vi "Img_Bird_eye_view.vi"(6 "parameters":T1={"P1"={"x"=970, "y"=485}, "P2"={"x"=0, "y"=750}, "Alfa"=6.0}, 8 "error in (no error)":errorcluster, 10 "Image Name":string="myimg", 11 "img annotation in":T2(plugin-control)) -> (0 "error out":errorcluster, 2 "img_corrected":T2(plugin-control), 3 "img annotation out":T2)   [LabVIEW 2021, in "Framework_lib.lvlib"]
uses:
  QMH/Framework_lib.lvlib
  <vilib>/vision/Image Controls.llb/IMAQ Image.ctl
  <vilib>/vision/NI_Vision_Development_Module.lvlib
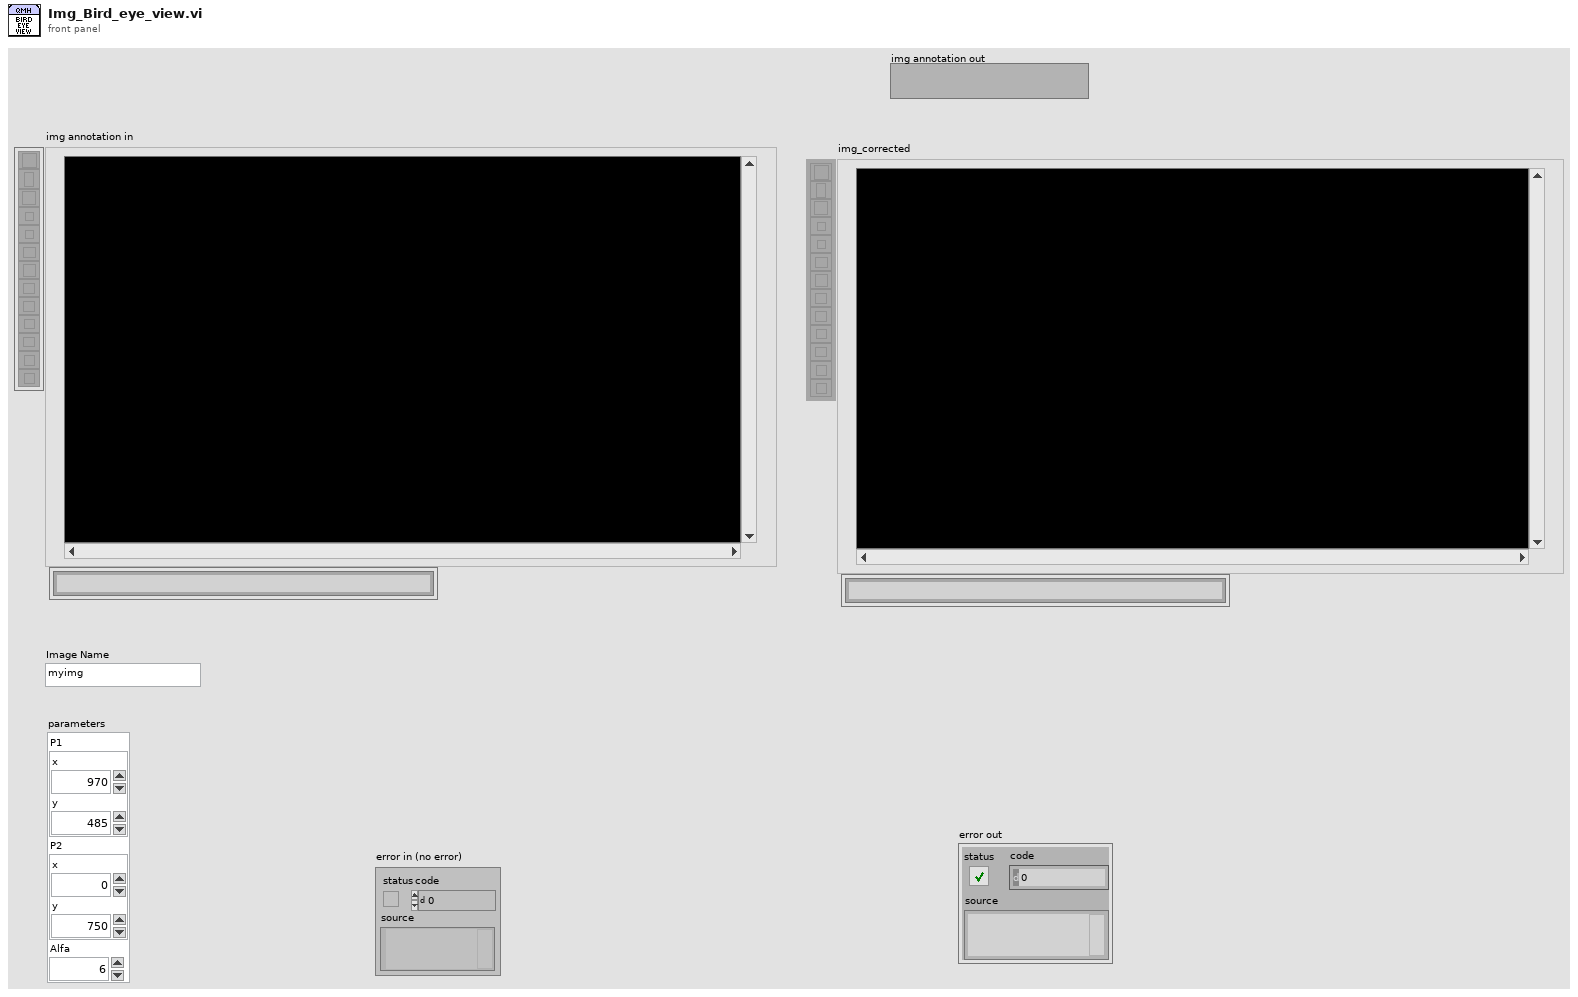
[diagram p1: front panel]
types:
  T1 = cluster{"P1":cluster{"x":i16, "y":i16}, "P2":cluster{"x":i16, "y":i16}, "Alfa":dbl}
  T2 = typedef "IMAQ Image.ctl" = refnum<image>
  T3 = typedef "Image Type" = u32
  T4 = enum32{"Zero Order", "Bilinear", "Quadratic", "Cubic", "Bilinear Fixed"}
  T5 = cluster{"Interpolation Type":enum32{"Zero Order", "Bilinear", "Quadratic", "Cubic", "Bilinear Fixed"}, "Destination Width":u32, "Destination Height":u32, "Fill Value":sgl}
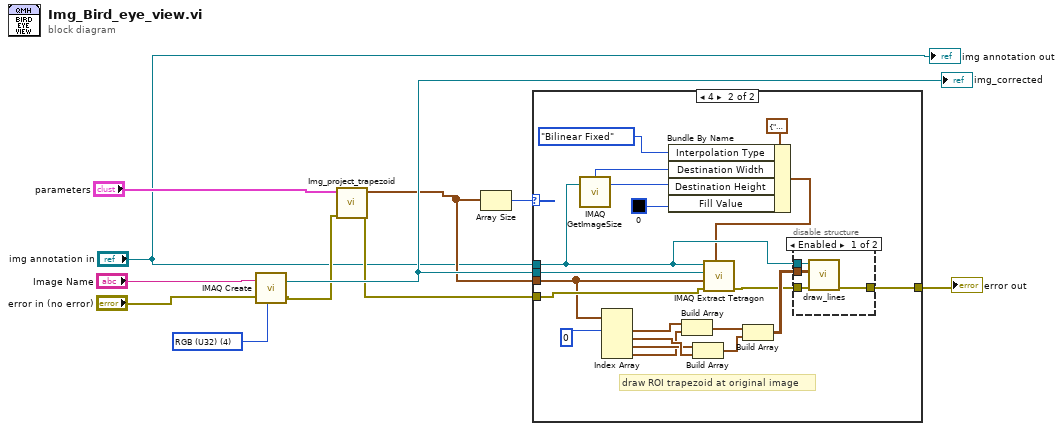
[diagram p0: block diagram]
diagram:
  w1 = T3 4 items=["Grayscale (U8)", "Grayscale (I16)", "Grayscale (SGL)", "Complex (CSG)", "RGB (U32)", "HSL (U32)", "RGB (U64)", "Grayscale (U16)"] ("Image Type")
  n1 = call "IMAQ Create"("Image Name"="Image Name", "Image Type"=w1, "error in (no error)"="error in (no error)") -> ("New Image"=w9:T2, "error out"=w8:errorcluster)  [unwired: 2 in]
  "img_corrected" <- w9
  n2 = call "Img_project_trapezoid.vi"("error in (no error)"=w8, "parameters"="parameters") -> ("error out"=w5:errorcluster, "trapezoid_ROI"=w7:cluster{"X":dbl, "Y":dbl}[])  [unwired: 8 in]
  n3 = Array Size(array=w7) -> (size(s)=w10:i32)
  n4 = case shown="4" w10 {
    tunnel: "img annotation in" -> [_ w19]
    tunnel: w9 -> [_ w32]
    tunnel: w7 -> [_ w20]
    tunnel: [w12 w22] -> w6
    tunnel: w5 -> [w12 w21]
    frame 0, Default {
    }
    frame 4 {
      # "draw ROI trapezoid at original image"
      n5 = call "IMAQ GetImageSize"("Image"=w19) -> ("Y Resolution"=w15:i32, "X Resolution"=w16:i32)  [unwired: 3 in, 1 out]
      n6 = Index Array(array=w20, index #1=0 ("index")) -> (element #1=w25:cluster{"X":dbl, "Y":dbl}, element #2=w28:cluster{"X":dbl, "Y":dbl}, element #3=w27:cluster{"X":dbl, "Y":dbl}, element #4=w26:cluster{"X":dbl, "Y":dbl})  [unwired: 3 in]
      n7 = Bundle By Name(cluster=T5 {"Interpolation Type"=enum."Zero Order", "Destination Width"=1920, "Destination Height"=1080, "Fill Value"=0.0} ("Options"), "Interpolation Type"=T4."Bilinear Fixed", "Destination Width"=w16, "Destination Height"=w15, "Fill Value"=u32 0) -> (w13:T5)
      n8 = Build Array(w25, w26) -> (w30:cluster{"X":dbl, "Y":dbl}[])
      n9 = Build Array(w27, w28) -> (w29:cluster{"X":dbl, "Y":dbl}[])
      n10 = call-poly "IMAQ Extract Tetragon"("Options"=w13, "error in (no error)"=w21, "Tetragon"=w20, "Image Dst"=w32, "Image Src"=w19) -> ("error out"=w23:errorcluster)  [unwired: 5 in, 1 out]
      n11 = Build Array(w30, w29) -> (w31:cluster{"X":dbl, "Y":dbl}[][])
      n12 = disable-structure shown="Enabled" {
        disable-tunnel: w31 -> [w36 _]
        disable-tunnel: w23 -> [w35 w37]
        disable-tunnel: [w34 w37] -> w22
        disable-tunnel: w19 -> [w33 _]
        frame Enabled {
          n13 = call "draw_lines.vi"("error in (no error)"=w35, "lines"=w36, "Image"=w33) -> ("error out"=w34:errorcluster)  [unwired: 7 in, 1 out]
        }
        frame Disabled {
        }
      }
    }
  }
  "error out" <- w6
  "img annotation out" <- "img annotation in"
